vi "SA Cond - Truncate ALL Signals.vi"(0 "wForm IN":waveform(dbl)[](array[waveform]), 5 "error in (no error)":errorcluster, 6 "Nb Signals":i32, 7 "Start (sec)":dbl, 8 "Anotate Signal Name":bool=TRUE, 9 "Duration (sec)":dbl=-1.0, 10 "Cut Option":T1(ring)) -> (11 "actual duration":dbl format="%0.2f", 13 "actual start samples/time":dbl format="%_8f", 14 "wForm OUT":waveform(dbl)[](array[waveform]), 19 "error out":errorcluster)   [LabVIEW 2022 SP3, in "GSwFormDSP.lvclass"]
uses:
  GSwFormDSP.lvclass
  Attribute List.ctl
  Attribute Options.ctl
  <vilib>/Waveform/WDTOps.llb/WDT Waveform Duration DBL.vi
  <vilib>/Waveform/WDTOps.llb/WDT Append Waveforms DBL.vi
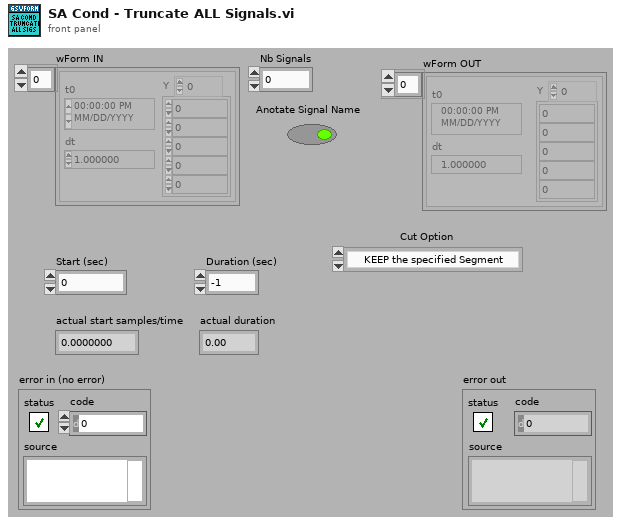
[diagram p1: front panel]
types:
  T1 = enum16{"KEEP the specified Segment", "DELETE the specified Segment"}
  T2 = typedef "GSwFormDSP.lvclass/Attribute Options.ctl" = enum16{"Append to Attribute using \"( )\"", "Replace Attribute Value"}
  T3 = typedef "GSwFormDSP.lvclass/Attribute List.ctl" = string
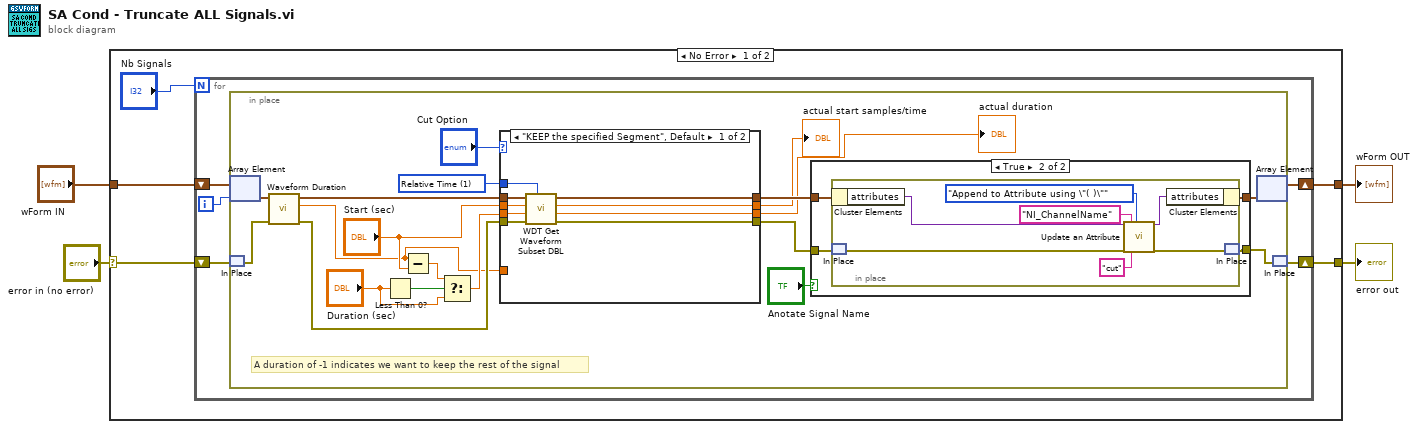
[diagram p0: block diagram]
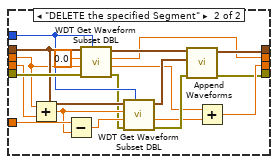
[diagram p2: hidden frame]
diagram:
  n1 = case shown="No Error" "error in (no error)" {
    selector: "error in (no error)" -> [w8 w76]
    tunnel: [w6 w76] -> w3
    tunnel: "wForm IN" -> [w9 w75]
    tunnel: [w7 w75] -> w1
    frame No Error {
      n2 = for {
        N: "Nb Signals" -> [_]
        shift-right: [w13] -> w7
        shift-left: w9 -> [w12]
        shift-right: [w10] -> w6
        shift-left: w8 -> [w11]
        i -> [w14]
        n3 = in-place {
          w33 = u16 1 items=["Samples", "Relative Time"] ("start/duration format")
          # "A duration of -1 indicates we want to keep the rest of the signal"
          n4 = in-place-array #1(w12, w14) -> (w27:waveform(dbl))
          n5 = in-place-match #2(w11) -> (w25:errorcluster)
          n6 = call-poly <vilib>:"Waveform Duration.vi"("error in (no error)"=w25, "waveform in"=w27) -> ("error out"=w24:errorcluster, "duration"=w15:dbl, "waveform out"=w26:waveform(dbl))  [unwired: 7 in]
          n7 = Less Than 0?(x="Duration (sec)") -> (x < 0?=w21:bool)
          n8 = Subtract(x=w15, y="Start (sec)") -> (x-y=w22:dbl)
          n9 = Select(t=w22, s=w21, f="Duration (sec)") -> (s? t:f=w19:dbl)
          n10 = case shown="\"KEEP the specified Segment\", Default" "Cut Option" {
            tunnel: w33 -> [w42 w58]
            tunnel: [w41 w48] -> w30
            tunnel: [w40 w43] -> w28
            tunnel: w26 -> [w39 w59]
            tunnel: w24 -> [w38 w61]
            tunnel: "Start (sec)" -> [w37 w56]
            tunnel: w19 -> [w36 w57]
            tunnel: [w35 w47] -> w18
            tunnel: [w34 w44] -> w17
            tunnel: w15 -> [_ w55]
            frame "KEEP the specified Segment", Default {
              n11 = call <vilib>:"WDT Get Waveform Subset DBL.vi"("start/duration format"=w42, "error in (no error)"=w38, "duration"=w36, "start samples/time"=w37, "waveform in"=w39) -> ("error out"=w40:errorcluster, "actual duration"=w34:dbl, "actual start samples/time"=w35:dbl, "waveform out"=w41:waveform(dbl))  [unwired: 1 in]
            }
            frame "DELETE the specified Segment" {
              n12 = Add(x=w56, y=w57) -> (x+y=w54:dbl)
              n13 = Subtract(x=w55, y=w54) -> (x-y=w53:dbl)
              n14 = call <vilib>:"WDT Get Waveform Subset DBL.vi"("start/duration format"=w58, "error in (no error)"=w61, "duration"=w56, "start samples/time"=0.0, "waveform in"=w59) -> ("error out"=w52:errorcluster, "actual duration"=w45:dbl, "actual start samples/time"=w47:dbl, "waveform out"=w51:waveform(dbl))  [unwired: 1 in]
              n15 = call <vilib>:"WDT Get Waveform Subset DBL.vi"("start/duration format"=w58, "error in (no error)"=w52, "duration"=w53, "start samples/time"=w54, "waveform in"=w59) -> ("error out"=w49:errorcluster, "actual duration"=w46:dbl, "waveform out"=w50:waveform(dbl))  [unwired: 1 in, 1 out]
              n16 = call-poly <vilib>:"Append Waveforms.vi"("error in (no error)"=w49, "waveform B"=w50, "waveform A"=w51) -> ("error out"=w43:errorcluster, "waveform out"=w48:waveform(dbl))  [unwired: 7 in]
              n17 = Add(x=w45, y=w46) -> (x+y=w44:dbl)
            }
          }
          "actual start samples/time" <- w18
          "actual duration" <- w17
          n18 = case shown="True" "Anotate Signal Name" {
            tunnel: [w63 w65] -> w31
            tunnel: w30 -> [w63 w67]
            tunnel: [w62 w64] -> w29
            tunnel: w28 -> [w62 w66]
            frame False {
            }
            frame True {
              n19 = in-place {
                n20 = in-place-cluster #3(w67) -> ("attributes"=w74:variant)
                n21 = in-place-match #4(w66) -> (w68:errorcluster)
                n22 = call "Update an Attribute.vi"("attributes in"=w74, "error in (no error)"=w68, "Attribute List"=T3 "NI_ChannelName", "Attribute Value"="cut" ("string"), "Attribute Option"=Attribute_Options."Append to Attribute using \"( )\"") -> ("attributes out"=w73:variant, "error out"=w72:errorcluster)  [unwired: 13 in]
                n23 = in-place-cluster #3("attributes"=w73) -> (w65:waveform(dbl))
                n24 = in-place-match #4(w72) -> (w64:errorcluster)
              }
            }
          }
          n25 = in-place-array #1(w31) -> (w13:waveform(dbl)[])  [unwired: 1 out]
          n26 = in-place-match #2(w29) -> (w10:errorcluster)
        }
      }
    }
    frame Error {
    }
  }
  "error out" <- w3
  "wForm OUT" <- w1
